vi "BumpSetpoint.vi"(8 "Bump Down Trigger":bool, 9 "Bump Up Trigger":bool, 10 "Bump Increment":dbl, 11 "Original Setpoint":dbl) -> (2 "Bumped Setpoint":dbl)   [LabVIEW 2019]
doc: "Bumps a setpoint up or down by a specified interval"
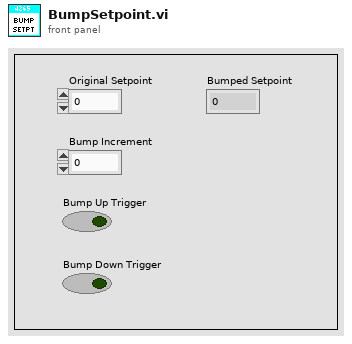
[diagram p1: front panel]
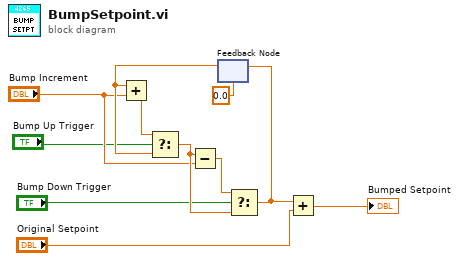
[diagram p0: block diagram]
diagram:
  n1 = feedback #1(0.0) -> (w9:dbl)
  n2 = Add(x=w9, y="Bump Increment") -> (x+y=w6:dbl)
  n3 = Select(t=w6, s="Bump Up Trigger", f=w9) -> (s? t:f=w10:dbl)
  n4 = Subtract(x=w10, y="Bump Increment") -> (x-y=w11:dbl)
  n5 = Select(t=w11, s="Bump Down Trigger", f=w10) -> (s? t:f=w5:dbl)
  n6 = feedback-in #1(w5) -> ()
  n7 = Add(x=w5, y="Original Setpoint") -> (x+y=→"Bumped Setpoint":dbl)
